vi "Output flag.vi"(9 "BKS_falilure":bool) -> (1 "Boolean 3":bool)   [LabVIEW 2016]
panel:
  out "Boolean":bool
  out "Boolean 2":bool
  in  "i>=20?":bool
  in  "=1?":bool
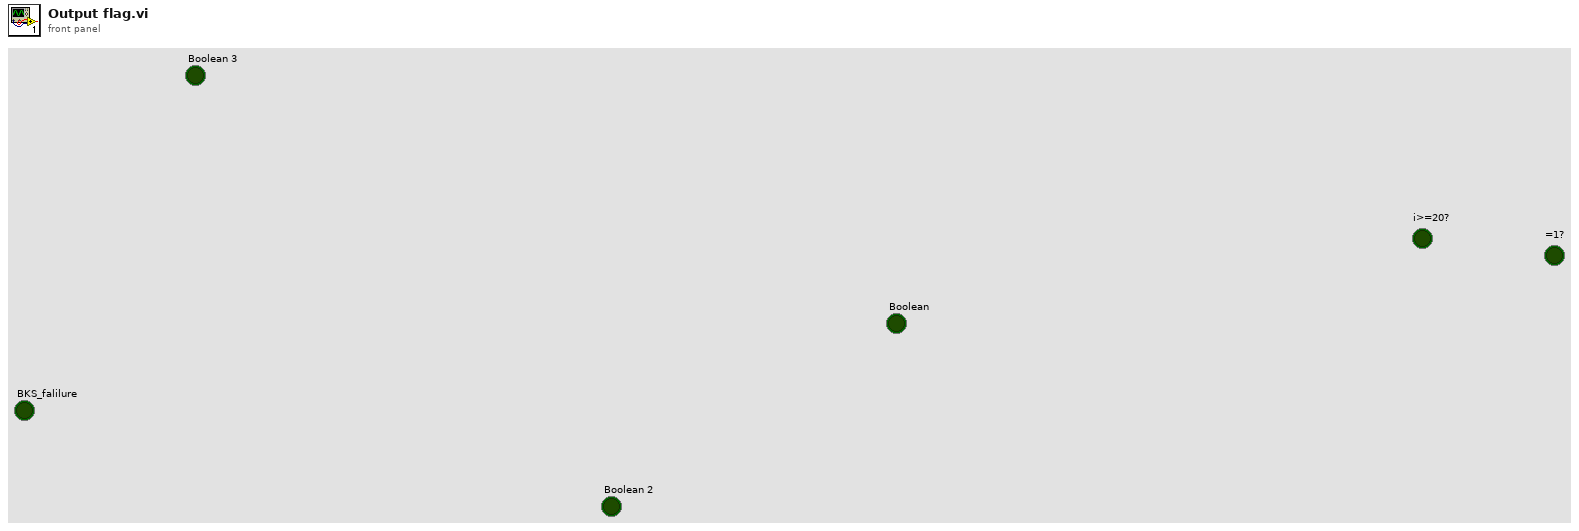
[diagram p1: front panel]
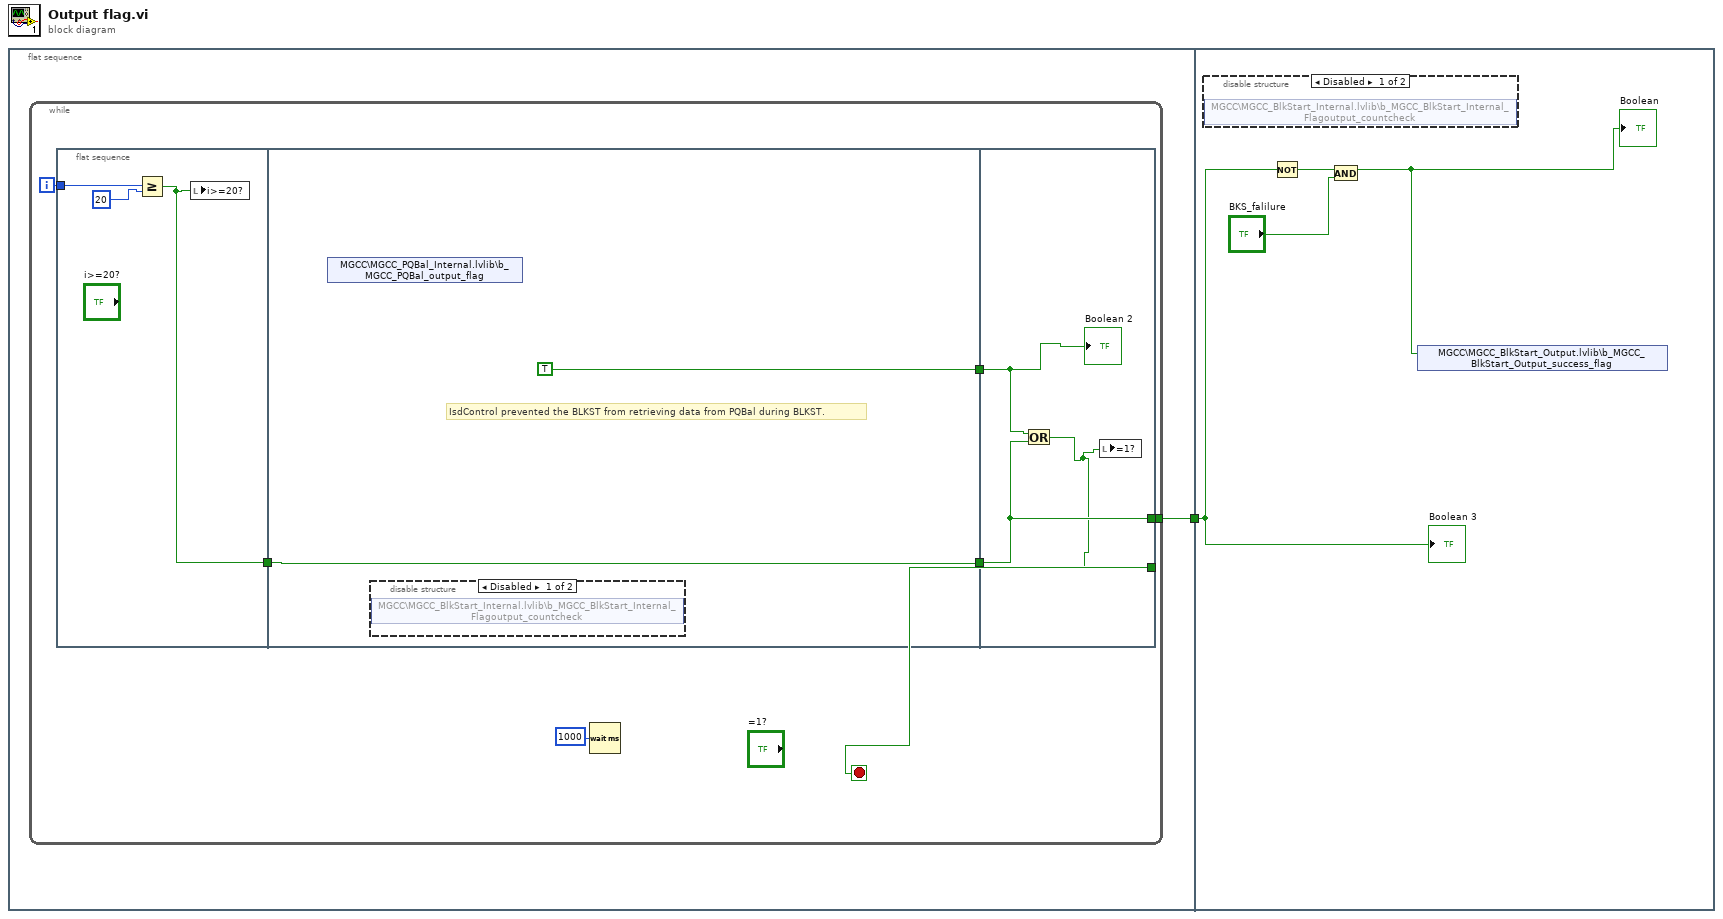
[diagram p0: block diagram]
diagram:
  n1 = flat-sequence {
    tunnel: [w2] -> w1
    tunnel: w1 -> [w20]
    frame #0 {
      n2 = while {
        tunnel: [w5] -> w2
        i -> [w8]
        stop <- w3 stop-if-true
        n3 = flat-sequence {
          tunnel: w8 -> [w12]
          tunnel: [w10] -> w4
          tunnel: [w14] -> w7
          tunnel: [TRUE ("Boolean")] -> w6
          tunnel: w4 -> [w14]
          tunnel: w7 -> [w16]
          tunnel: w6 -> [w17]
          tunnel: [w16] -> w5
          tunnel: [w15] -> w3
          frame #0 {
            n4 = Greater Or Equal?(x=w12, y=20) -> (x >= y?=w10:bool)
            n5 = local write "i>=20?"(w10) -> ()
          }
          frame #1 {
            # "IsdControl prevented the BLKST from retrieving data from PQBal during BLKST."
            n6 = shared-variable "MGCC\\MGCC_PQBal_Internal.lvlib\\b_MGCC_PQBal_output_flag"() -> ()  [unwired: 1 in, 2 out]
            n7 = disable-structure shown="Disabled" {
              frame Disabled {
                n8 = shared-variable "MGCC\\MGCC_BlkStart_Internal.lvlib\\b_MGCC_BlkStart_Internal_Flagoutput_countcheck"() -> ()  [unwired: 2 in, 1 out]
              }
              frame Enabled {
              }
            }
          }
          frame #2 {
            n9 = Or(x=w17, y=w16) -> (x .or. y?=w15:bool)
            n10 = local write "=1?"(w15) -> ()
            "Boolean 2" <- w17
          }
        }
        n11 = Wait (ms)(milliseconds to wait=1000) -> ()  [unwired: 1 out]
      }
    }
    frame #1 {
      n12 = disable-structure shown="Disabled" {
        frame Disabled {
          n13 = shared-variable "MGCC\\MGCC_BlkStart_Internal.lvlib\\b_MGCC_BlkStart_Internal_Flagoutput_countcheck"() -> ()  [unwired: 1 in, 2 out]
        }
        frame Enabled {
        }
      }
      n14 = Not(x=w20) -> (.not. x?=w21:bool)
      n15 = And(x=w21, y="BKS_falilure") -> (x .and. y?=w19:bool)
      "Boolean" <- w19
      n16 = shared-variable "MGCC\\MGCC_BlkStart_Output.lvlib\\b_MGCC_BlkStart_Output_success_flag"(w19) -> ()  [unwired: 1 in, 1 out]
      "Boolean 3" <- w20
    }
  }
